vi "Save Report to File.vi"(0 "report in":refnum<class "NI_HTML.lvclass">, 5 "report file path":path, 7 "prompt to replace? (F)":bool, 9 "password (\"\")":string, 11 "error in (no error)":errorcluster) -> (4 "report out":refnum<class "NI_HTML.lvclass">, 15 "error out":errorcluster)   [LabVIEW 2015, in "NI_HTML.lvclass"]
doc: "Saves an HTML, Word, or Excel report to the file specified in <B>report file path</B>. You cannot use this VI with standard reports."
uses:
  <vilib>/Utility/NIReport.llb/HTML/NI_HTML.lvclass
  <vilib>/Utility/NIReport.llb/HTML/NI_HTML.lvclass/NI_HTML.ctl
  <vilib>/Utility/NIReport.llb/NI_ReportGenerationCore.lvlib
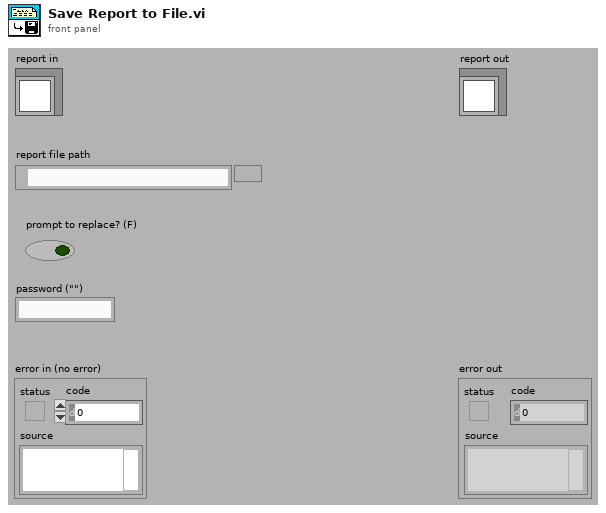
[diagram p1: front panel]
types:
  T1 = enum16{"open", "replace", "create", "open or create", "replace or create", "replace or create with confirmation"}
  T2 = typedef "NI_ReportGenerationCore.lvlib/HTML Report Data.ctl" = cluster{"Body Text":string, "Font Tag":string, "Title Text":string, "Header Text":string, "Footer Text":string, "Image List":path[]}
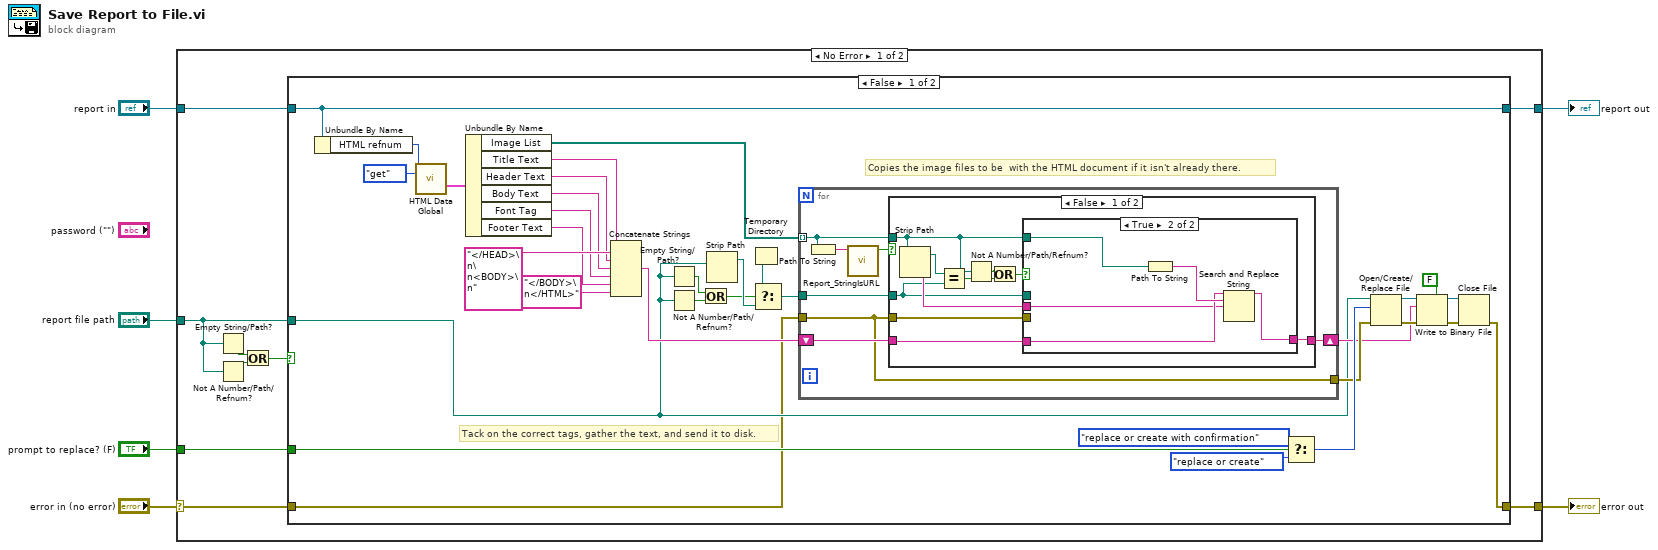
[diagram p0: block diagram]
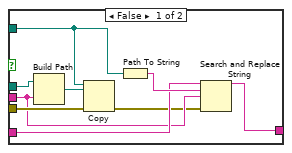
[diagram p2: hidden frame]
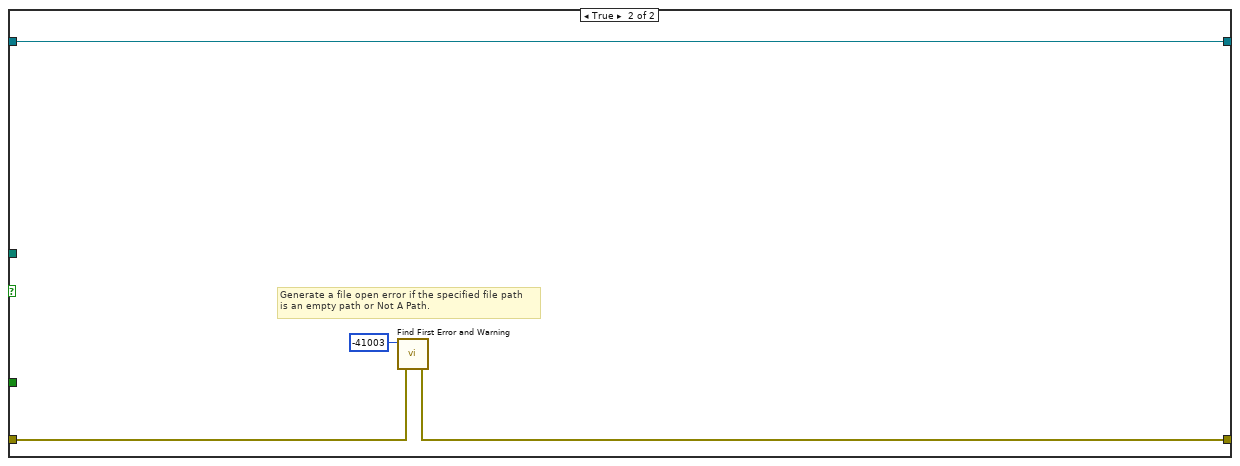
[diagram p4: hidden frame]
diagram:
  n1 = case shown="No Error" "error in (no error)" {
    selector: "error in (no error)" -> [w9 w86]
    tunnel: [w10 w85] -> w4
    tunnel: "report in" -> [w11 w85]
    tunnel: "report file path" -> [w12 _]
    tunnel: [w8 w86] -> w2
    tunnel: "prompt to replace? (F)" -> [w7 _]
    frame No Error {
      n2 = Empty String/Path?(string/path=w12) -> (empty?=w14:bool)
      n3 = Not A Number/Path/Refnum?(number/path/refnum=w12) -> (NaN/Path/Refnum?=w13:bool)
      n4 = Or(x=w14, y=w13) -> (x .or. y?=w15:bool)
      n5 = case shown="False" w15 {
        tunnel: [w17 w84] -> w10
        tunnel: w11 -> [w17 w84]
        tunnel: w12 -> [w25 _]
        tunnel: w9 -> [w23 w82]
        tunnel: [w22 w81] -> w8
        tunnel: w7 -> [w24 _]
        frame False {
          # "Copies the image files to be  with the HTML document if it isn't already there."
          # "Tack on the correct tags, gather the text, and send it to disk."
          n6 = Unbundle By Name(w17) -> ("HTML refnum"=w21:u32)
          n7 = call <vilib>:"HTML Data Global.vi"("HTML refnum"=w21, "menu"=enum16{"init", "get", "set", "delete"}."get") -> ("HTML report data out"=w19:T2)  [unwired: 1 in, 12 out]
          n8 = Unbundle By Name(w19) -> ("Image List"=w18:path[], "Title Text"=w27:string, "Header Text"=w28:string, "Body Text"=w29:string, "Font Tag"=w26:string, "Footer Text"=w32:string)
          n9 = Concatenate Strings(w27, "</HEAD>\n\n<BODY>\n" ("Substring"), w28, w29, w26, w32, "</BODY>\n</HTML>") -> (w38:string)
          n10 = Empty String/Path?(string/path=w25) -> (empty?=w35:bool)
          n11 = Not A Number/Path/Refnum?(number/path/refnum=w25) -> (NaN/Path/Refnum?=w34:bool)
          n12 = Or(x=w35, y=w34) -> (x .or. y?=w16:bool)
          n13 = Strip Path(path=w25) -> (stripped path=w36:path)  [unwired: 1 out]
          n14 = Temporary Directory() -> (w37:path)
          n15 = Select(t=w37, s=w16, f=w36) -> (s? t:f=w30:path)
          n16 = for {
            tunnel: w30 -> [w52]
            tunnel: w23 -> [w53]
            tunnel: [w53] -> w47
            tunnel: w18 -> [w50] mode=indexing
            shift-right: [w55] -> w39
            shift-left: w38 -> [w54]
            n17 = Path To String(path=w50) -> (string=w49:string)
            n18 = call <vilib>:"Report_StringIsURL.vi"("String"=w49) -> ("Is URL?"=w51:bool)  [unwired: 1 in, 9 out]
            n19 = case shown="False" w51 {
              tunnel: [w63 w80] -> w55
              tunnel: w54 -> [w62 w80]
              tunnel: w53 -> [w61 _]
              tunnel: w52 -> [w59 _]
              tunnel: w50 -> [w57 _]
              frame False {
                n20 = Strip Path(path=w57) -> (stripped path=w56:path, name=w60:string)
                n21 = Equal?(x=w56, y=w59) -> (x = y?=w65:bool)
                n22 = Not A Number/Path/Refnum?(number/path/refnum=w57) -> (NaN/Path/Refnum?=w64:bool)
                n23 = Or(x=w64, y=w65) -> (x .or. y?=w58:bool)
                n24 = case shown="True" w58 {
                  tunnel: w59 -> [w71 _]
                  tunnel: w61 -> [w74 _]
                  tunnel: w57 -> [w67 w76]
                  tunnel: w62 -> [w69 w78]
                  tunnel: [w72 w77] -> w63
                  tunnel: w60 -> [w68 w75]
                  frame False {
                    n25 = Build Path(base path=w71, name or relative path=w68) -> (appended path=w70:path)
                    n26 = Copy(8:w74, 10:w70, 11:w67) -> (0:w66:errorcluster)  [unwired: 4 out]
                    n27 = Path To String(path=w67) -> (string=w73:string)
                    n28 = Search and Replace String(input string=w69, search string=w73, replace string=w68, error in=w66) -> (result string=w72:string)  [unwired: 7 out]
                  }
                  frame True {
                    n29 = Path To String(path=w76) -> (string=w79:string)
                    n30 = Search and Replace String(input string=w78, search string=w79, replace string=w75) -> (result string=w77:string)  [unwired: 1 in, 7 out]
                  }
                }
              }
              frame True {
              }
            }
          }
          n31 = Select(t=T1."replace or create with confirmation" ("operation (0:open)"), s=w24, f=T1."replace or create" ("operation (0:open)")) -> (s? t:f=w48:T1)
          n32 = Open/Create/Replace File(file path (use dialog)=w25, error in=w47, operation (0:open)=w48) -> (refnum out=w45:refnum<file>, error out=w46:errorcluster)  [unwired: 4 out]
          n33 = Write to Binary File(file (use dialog)=w45, data=w39, error in=w46, 5:FALSE ("prepend array or string size? (T)")) -> (refnum out=w40:refnum<file>, error out=w41:errorcluster)  [unwired: 3 out]
          n34 = Close File(refnum=w40, error in=w41) -> (error out=w22:errorcluster)  [unwired: 1 out]
        }
        frame True {
          # "Generate a file open error if the specified file path\nis an empty path or Not A Path."
          n35 = call <vilib>:"Find First Error and Warning.vi"("error in (no error)"=w82, "error code"=-41003) -> ("error out"=w81:errorcluster)  [unwired: 1 in, 4 out]
        }
      }
    }
    frame Error {
    }
  }
  "error out" <- w2
  "report out" <- w4
